vi "GEMM_Only(CuLab).vi"() -> ()   [LabVIEW 2020]
doc: "Solves the heat equation in a two-dimensional area using a Finite Element Method."
uses:
  <vilib>/Ngene/CuLab - GPU Accelerated Toolkit/Toolkit/Low_Level/Tensor_Classes/T_Children/T2D/T2D_Children/T2D_SGL/Create_Push.vi
  <vilib>/Ngene/CuLab - GPU Accelerated Toolkit/Toolkit/API/Array/Initialize Array/T1D/CU_Initialize Array_T1D_SGL.vi
  <vilib>/Ngene/CuLab - GPU Accelerated Toolkit/Toolkit/API/Linear Algebra/BLAS2/gemv/CU_gemv/CU_Sgemv.vi
  <vilib>/Ngene/CuLab - GPU Accelerated Toolkit/Toolkit/Low_Level/Tensor_Classes/T_Children/T1D/T1D_Children/T1D_SGL/Pull.vi
  subVIs/Heat Equation Solver.lvlib
  <vilib>/Ngene/CuLab - GPU Accelerated Toolkit/Toolkit/CuLab.lvlib
  <vilib>/ptbypt/NI_PtbyPt.lvlib
  <vilib>/Ngene/CuLab - GPU Accelerated Toolkit/Toolkit/Low_Level/Tensor_Classes/T_Children/T2D/T2D_Children/T2D_SGL/T2D_SGL.lvclass
  <vilib>/Ngene/CuLab - GPU Accelerated Toolkit/Toolkit/Low_Level/Tensor_Classes/T_Children/T1D/T1D_Children/T1D_SGL/T1D_SGL.lvclass
panel:
  out "stop display":bool
  out "Z Graph":sgl[](array[numeric])
  out "time":dbl[unit] format="%#_4p"
  out "time graph":dbl(graph)
  out "Error out":errorcluster
  in  "stop":bool
  # "GEMM based on CuLab"
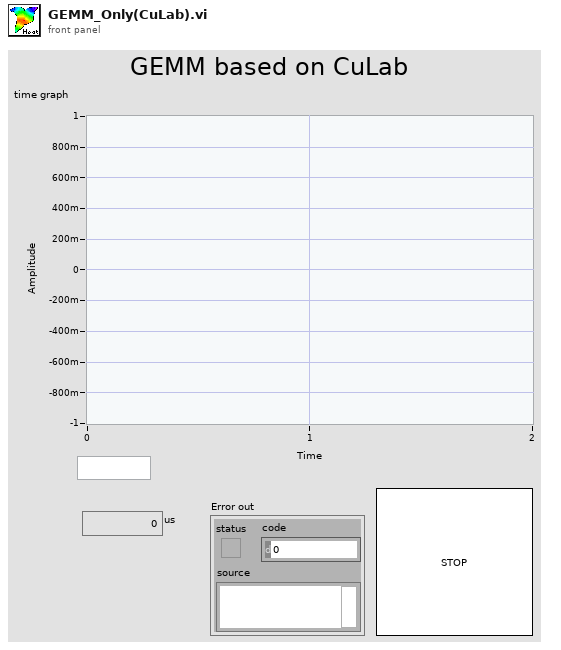
[diagram p1: front panel]
types:
  T1 = typedef "NI_Matrix.lvlib/RealMatrix.ctl" = dbl[][]
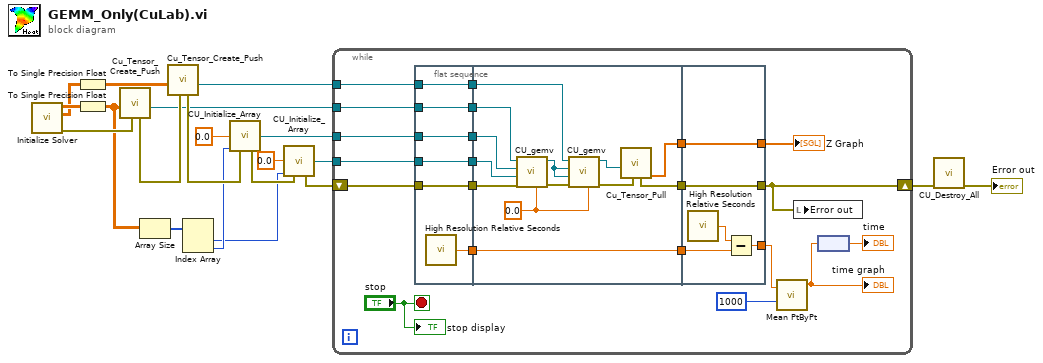
[diagram p0: block diagram]
diagram:
  n1 = call "Initialize Solver.vi"() -> ("error out"=w19:errorcluster, "Mass"=w9:T1, "Stiffness"=w13:T1)  [unwired: 8 in, 1 out]
  n2 = To Single Precision Float(number=w9) -> (single precision float=w7:sgl[][])
  n3 = To Single Precision Float(number=w13) -> (single precision float=w8:sgl[][])
  n4 = call-poly <vilib>:"Cu_Tensor_Create_Push.vi"("error in (no error)"=w19, "CPU_Data_2D_SGL"=w8) -> ("T2D_SGL out"=w15:refnum<class "T2D_SGL.lvclass">, "error out"=w20:errorcluster)  [unwired: 8 in]
  n5 = Array Size(array=w8) -> (size(s)=w12:i32[])
  n6 = call-poly <vilib>:"Cu_Tensor_Create_Push.vi"("error in (no error)"=w20, "CPU_Data_2D_SGL"=w7) -> ("T2D_SGL out"=w14:refnum<class "T2D_SGL.lvclass">, "error out"=w17:errorcluster)  [unwired: 8 in]
  n7 = Index Array(array=w12) -> (element #1=w2:i32, element #2=w10:i32)  [unwired: 2 in]
  n8 = call-poly <vilib>:"CU_Initialize_Array.vi"("element"=sgl 0.0 ("SGL"), "dimension size"=w10, "error in (no error)"=w17) -> ("initialized Tensor"=w11:refnum<class "T1D_SGL.lvclass">, "error out"=w5:errorcluster)  [unwired: 11 in]
  n9 = call-poly <vilib>:"CU_Initialize_Array.vi"("element"=sgl 0.0 ("SGL"), "dimension size"=w2, "error in (no error)"=w5) -> ("initialized Tensor"=w6:refnum<class "T1D_SGL.lvclass">, "error out"=w18:errorcluster)  [unwired: 11 in]
  n10 = while {
    shift-right: [w29] -> w16
    shift-left: w18 -> [w30]
    tunnel: w14 -> [w36]
    tunnel: w15 -> [w35]
    tunnel: w11 -> [w33]
    tunnel: w6 -> [w27]
    stop <- "stop" stop-if-true
    n11 = flat-sequence {
      tunnel: w36 -> [w46]
      tunnel: w35 -> [w47]
      tunnel: [w47] -> w41
      tunnel: [w46] -> w40
      tunnel: [w45] -> w39
      tunnel: [w44] -> w34
      tunnel: w33 -> [w44]
      tunnel: [w43] -> w32
      tunnel: w30 -> [w43]
      tunnel: [w42] -> w28
      tunnel: w27 -> [w42]
      tunnel: w41 -> [w57]
      tunnel: w40 -> [w48]
      tunnel: w39 -> [w59]
      tunnel: [w59] -> w38
      tunnel: w34 -> [w51]
      tunnel: w32 -> [w58]
      tunnel: [w60] -> w31
      tunnel: w28 -> [w54]
      tunnel: [w55] -> w26
      tunnel: w38 -> [w65]
      tunnel: w31 -> [w63]
      tunnel: [w63] -> w29
      tunnel: [w62] -> w21
      tunnel: w26 -> [w62]
      tunnel: [w61] -> w23
      frame #0 {
        n12 = call <vilib>:"High Resolution Relative Seconds.vi"() -> ("relative seconds"=w45:dbl)
      }
      frame #1 {
        w50 = sgl 0.0 ("beta")
        n13 = call-poly <vilib>:"CU_gemv.vi"("beta"=w50, "error in (no error)"=w58, "y"=w54, "x"=w51, "A"=w57) -> ("error out"=w56:errorcluster, "y out"=w49:refnum<class "T1D_SGL.lvclass">)  [unwired: 5 in]
        n14 = call-poly <vilib>:"CU_gemv.vi"("beta"=w50, "error in (no error)"=w56, "y"=w49, "x"=w49, "A"=w48) -> ("error out"=w52:errorcluster, "y out"=w53:refnum<class "T1D_SGL.lvclass">)  [unwired: 5 in]
        n15 = call-poly <vilib>:"Cu_Tensor_Pull.vi"("error in (no error)"=w52, "T1D_SGL in"=w53) -> ("Dest out"=w55:sgl[], "error out"=w60:errorcluster)  [unwired: 7 in, 1 out]
      }
      frame #2 {
        n16 = call <vilib>:"High Resolution Relative Seconds.vi"() -> ("relative seconds"=w64:dbl)
        n17 = Subtract(x=w64, y=w65) -> (x-y=w61:dbl)
      }
    }
    n18 = call <vilib>:"Mean PtByPt.vi"("x"=w23, "sample length"=1000) -> ("mean"=w24:dbl)  [unwired: 2 in, 1 out]
    "time graph" <- w24
    n19 = local write "Error out"(w29) -> ()
    n20 = node(w24) -> (→"time":dbl[unit])
    "Z Graph" <- w21
    "stop display" <- "stop"
  }
  n21 = call <vilib>:"CU_Destroy_All.vi"("error in"=w16) -> ("error out"=→"Error out":errorcluster)  [unwired: 10 in]
